vi "ChannelListToNumChannels.vi"(11 "Channels":T1) -> (3 "Numeric":i32)   [LabVIEW 2016, in "DAQ.lvclass"]
uses:
  DAQ.lvclass
  Typedefs/PrivateEvents--DAQ.AI.Channels.ctl
  <vilib>/regexp/Match Regular Expression.xnode
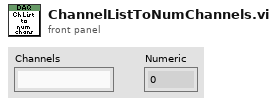
[diagram p1: front panel]
types:
  T1 = typedef "PrivateEvents--DAQ.AI.Channels.ctl" = string
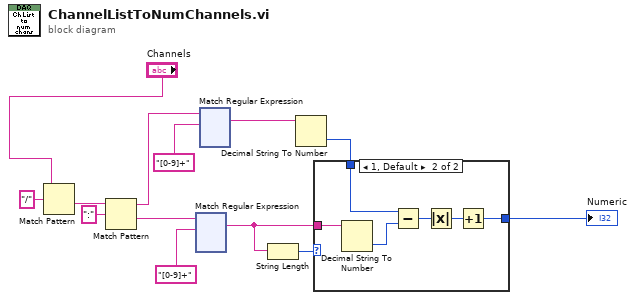
[diagram p0: block diagram]
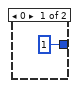
[diagram p2: hidden frame]
diagram:
  n1 = Match Pattern(string="Channels", regular expression="/") -> (after substring=w3:T1)  [unwired: 1 in, 3 out]
  n2 = Match Pattern(string=w3, regular expression=":") -> (before substring=w8:T1, after substring=w7:T1)  [unwired: 1 in, 2 out]
  n3 = xnode "Match Regular Expression"("input string"=w7, "regular expression"="[0-9]+") -> ("whole match"=w10:string)  [unwired: 4 in, 4 out]
  n4 = xnode "Match Regular Expression"("input string"=w8, "regular expression"="[0-9]+") -> ("whole match"=w5:string)  [unwired: 4 in, 4 out]
  n5 = String Length(string=w10) -> (length=w11:i32)
  n6 = Decimal String To Number(string=w5) -> (number=w6:i32)  [unwired: 2 in, 1 out]
  n7 = case shown="1, Default" w11 {
    tunnel: w6 -> [_ w20]
    tunnel: [1 w16] -> w13
    tunnel: w10 -> [_ w15]
    frame 0 {
    }
    frame 1, Default {
      n8 = Decimal String To Number(string=w15) -> (number=w19:i32)  [unwired: 2 in, 1 out]
      n9 = Subtract(x=w20, y=w19) -> (x-y=w18:i32)
      n10 = Absolute Value(x=w18) -> (abs(x)=w17:i32)
      n11 = Increment(x=w17) -> (x+1=w16:i32)
    }
  }
  "Numeric" <- w13
